vi "Example All Data.vi"() -> ()   [LabVIEW 2010]
uses:
  C:/tf/play/labview/Tinkerforge.dll
  Tinkerforge.dll
panel:
  out "calibration status":u8
  out "temperature (°C)":i16
  out "gravity vector (m/s²)":sgl[](array[numeric])
  out "linear acceleration (m/s²)":sgl[](array[numeric])
  out "euler angle (°)":sgl[](array[numeric])
  out "angular velocity (°/s)":sgl[](array[numeric])
  out "magnetic field (µT)":sgl[](array[numeric])
  out "quaternion":sgl[](array[numeric])
  out "acceleration (m/s²)":sgl[](array[numeric]) format="%.2f"
  in  "stop":bool
  in  "uid":string="Ron"
  in  "port":i32=4223
  in  "host":string="localhost"
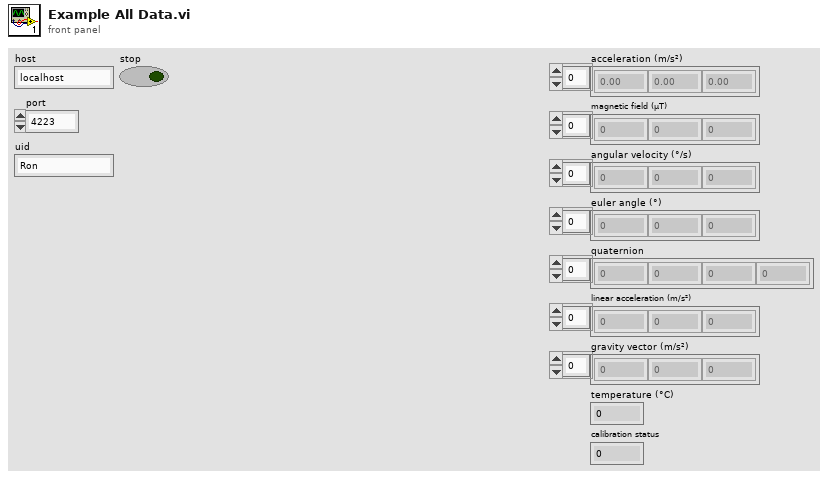
[diagram p1: front panel]
types:
  T1 = cluster{"acceleration":i16[], "magneticField":i16[], "angularVelocity":i16[], "eulerAngle":i16[], "quaternion":i16[], "linearAcceleration":i16[], "gravityVector":i16[], "temperature":i16, "calibrationStatus":u8}
  T2 = cluster{"acceleration[0]":i16, "acceleration[1]":i16, "acceleration[2]":i16, "acceleration[3]":i16, "acceleration[4]":i16, "acceleration[5]":i16, "acceleration[6]":i16, "acceleration[7]":i16, "acceleration[8]":i16}
  T3 = cluster{"magneticField[0]":i16, "magneticField[1]":i16, "magneticField[2]":i16, "magneticField[3]":i16, "magneticField[4]":i16, "magneticField[5]":i16, "magneticField[6]":i16, "magneticField[7]":i16, "magneticField[8]":i16}
  T4 = cluster{"angularVelocity[0]":i16, "angularVelocity[1]":i16, "angularVelocity[2]":i16, "angularVelocity[3]":i16, "angularVelocity[4]":i16, "angularVelocity[5]":i16, "angularVelocity[6]":i16, "angularVelocity[7]":i16, "angularVelocity[8]":i16}
  T5 = cluster{"eulerAngle[0]":i16, "eulerAngle[1]":i16, "eulerAngle[2]":i16, "eulerAngle[3]":i16, "eulerAngle[4]":i16, "eulerAngle[5]":i16, "eulerAngle[6]":i16, "eulerAngle[7]":i16, "eulerAngle[8]":i16}
  T6 = cluster{"quaternion[0]":i16, "quaternion[1]":i16, "quaternion[2]":i16, "quaternion[3]":i16, "quaternion[4]":i16, "quaternion[5]":i16, "quaternion[6]":i16, "quaternion[7]":i16, "quaternion[8]":i16}
  T7 = cluster{"linearAcceleration[0]":i16, "linearAcceleration[1]":i16, "linearAcceleration[2]":i16, "linearAcceleration[3]":i16, "linearAcceleration[4]":i16, "linearAcceleration[5]":i16, "linearAcceleration[6]":i16, "linearAcceleration[7]":i16, "linearAcceleration[8]":i16}
  T8 = cluster{"gravityVector[0]":i16, "gravityVector[1]":i16, "gravityVector[2]":i16, "gravityVector[3]":i16, "gravityVector[4]":i16, "gravityVector[5]":i16, "gravityVector[6]":i16, "gravityVector[7]":i16, "gravityVector[8]":i16}
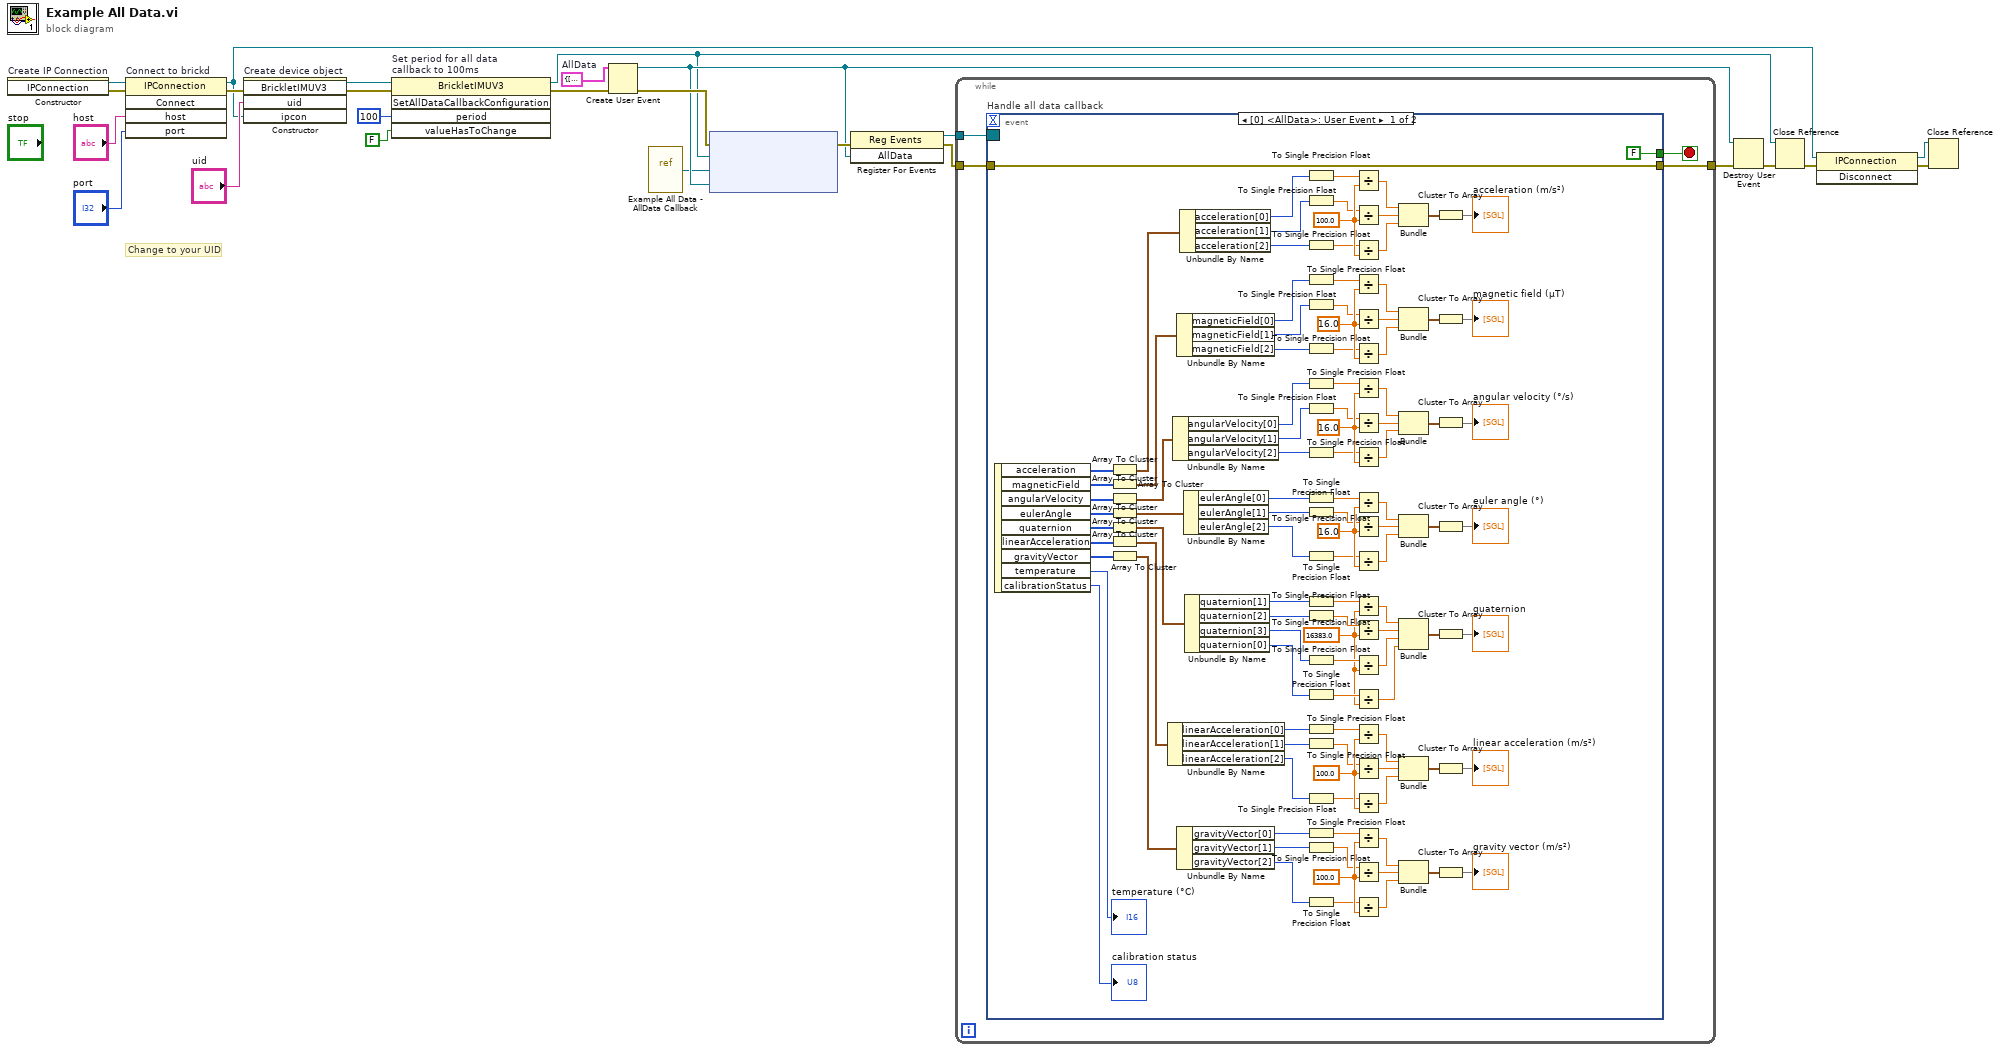
[diagram p0: block diagram]
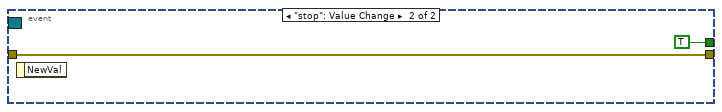
[diagram p2: hidden frame]
diagram:
  w9 = T1 {"acceleration"=[], "magneticField"=[], "angularVelocity"=[], "eulerAngle"=[], "quaternion"=[], "linearAcceleration"=[], "gravityVector"=[], "temperature"=0, "calibrationStatus"=0}  # AllData
  # "Change to your UID"
  n1 = constructor on="Create IP Connection" class="IPConnection"() -> (reference out=w25:refnum<k24>, error out=w3:errorcluster)  [unwired: 3 in, 1 out]
  n2 = invoke on="Connect to brickd" class="IPConnection" method="Connect"(reference=w25, error in=w3, "host"="host", "port"="port") -> (reference out=w18:refnum<k24>, error out=w21:errorcluster)  [unwired: 1 in, 3 out]
  n3 = constructor on="Create device object" class="BrickletIMUV3"(error in=w21, "uid"="uid", "ipcon"=w18) -> (reference out=w6:refnum<k24>, error out=w8:errorcluster)  [unwired: 2 in, 3 out]
  n4 = invoke on="Set period for all data\ncallback to 100ms" class="BrickletIMUV3" method="SetAllDataCallbackConfiguration"(reference=w6, error in=w8, "period"=i64 100, "valueHasToChange"=FALSE) -> (reference out=w5:refnum<k24>, error out=w7:errorcluster)  [unwired: 1 in, 3 out]
  n5 = Create User Event(user event datatype=w9, error in=w7) -> (user event=w11:refnum<user-event>, error out=w16:errorcluster)
  n6 = vi-ref "Example All Data - AllData Callback.vi"() -> ("vi reference"=w1:refnum<vi>)
  n7 = node ("Register Event Callback")(w16, w5, w1, w11) -> (w15:errorcluster)  [unwired: 1 in, 1 out]
  n8 = register-events(error in=w15, w11) -> (reference out=w14:refnum<event-registration>, error out=w12:errorcluster)  [unwired: 1 in]
  n9 = while {
    tunnel: w14 -> [w29]
    tunnel: [w28] -> w13
    tunnel: w12 -> [w27]
    stop <- w26 stop-if-true
    n10 = event "Handle all data callback" shown="[0] <AllData>: User Event" {
      selector: w29 -> [_ _]
      dyn-events: _ -> [_ _]
      timeout: _ -> [_ _]
      tunnel: [w134 w135] -> w28
      tunnel: w27 -> [w134 w135]
      tunnel: [FALSE TRUE] -> w26
      event User Event {
        w38 = sgl 100.0 ("y")
        w52 = sgl 100.0 ("y")
        w66 = sgl 16.0 ("y")
        w80 = sgl 16.0 ("y")
        w94 = sgl 16.0 ("y")
        w103 = sgl 16383.0 ("y")
        w123 = sgl 100.0 ("y")
        n11 = event-data() -> ("acceleration"=w132:i16[], "magneticField"=w89:i16[], "angularVelocity"=w75:i16[], "eulerAngle"=w60:i16[], "quaternion"=w107:i16[], "linearAcceleration"=w47:i16[], "gravityVector"=w33:i16[], "temperature"=→"temperature (°C)":i16, "calibrationStatus"=→"calibration status":u8)  [unwired: 1 in]
        n12 = Array To Cluster(array=w132) -> (cluster=w131:T2)
        n13 = Array To Cluster(array=w89) -> (cluster=w101:T3)
        n14 = Array To Cluster(array=w75) -> (cluster=w87:T4)
        n15 = Array To Cluster(array=w60) -> (cluster=w73:T5)
        n16 = Array To Cluster(array=w107) -> (cluster=w118:T6)
        n17 = Array To Cluster(array=w47) -> (cluster=w59:T7)
        n18 = Array To Cluster(array=w33) -> (cluster=w45:T8)
        n19 = Unbundle By Name(w59) -> ("linearAcceleration[0]"=w54:i16, "linearAcceleration[1]"=w51:i16, "linearAcceleration[2]"=w50:i16)
        n20 = Unbundle By Name(w87) -> ("angularVelocity[0]"=w82:i16, "angularVelocity[1]"=w79:i16, "angularVelocity[2]"=w78:i16)
        n21 = Unbundle By Name(w101) -> ("magneticField[0]"=w96:i16, "magneticField[1]"=w93:i16, "magneticField[2]"=w92:i16)
        n22 = Unbundle By Name(w45) -> ("gravityVector[0]"=w40:i16, "gravityVector[1]"=w37:i16, "gravityVector[2]"=w36:i16)
        n23 = Unbundle By Name(w131) -> ("acceleration[0]"=w125:i16, "acceleration[1]"=w122:i16, "acceleration[2]"=w121:i16)
        n24 = Unbundle By Name(w73) -> ("eulerAngle[0]"=w68:i16, "eulerAngle[1]"=w65:i16, "eulerAngle[2]"=w64:i16)
        n25 = Unbundle By Name(w118) -> ("quaternion[1]"=w113:i16, "quaternion[2]"=w111:i16, "quaternion[3]"=w110:i16, "quaternion[0]"=w104:i16)
        n26 = To Single Precision Float(number=w125) -> (single precision float=w124:sgl)
        n27 = To Single Precision Float(number=w122) -> (single precision float=w120:sgl)
        n28 = To Single Precision Float(number=w121) -> (single precision float=w119:sgl)
        n29 = To Single Precision Float(number=w96) -> (single precision float=w95:sgl)
        n30 = To Single Precision Float(number=w93) -> (single precision float=w91:sgl)
        n31 = To Single Precision Float(number=w92) -> (single precision float=w90:sgl)
        n32 = To Single Precision Float(number=w82) -> (single precision float=w81:sgl)
        n33 = To Single Precision Float(number=w79) -> (single precision float=w77:sgl)
        n34 = To Single Precision Float(number=w78) -> (single precision float=w76:sgl)
        n35 = To Single Precision Float(number=w68) -> (single precision float=w67:sgl)
        n36 = To Single Precision Float(number=w65) -> (single precision float=w63:sgl)
        n37 = To Single Precision Float(number=w64) -> (single precision float=w62:sgl)
        n38 = To Single Precision Float(number=w113) -> (single precision float=w112:sgl)
        n39 = To Single Precision Float(number=w111) -> (single precision float=w109:sgl)
        n40 = To Single Precision Float(number=w110) -> (single precision float=w108:sgl)
        n41 = To Single Precision Float(number=w104) -> (single precision float=w106:sgl)
        n42 = To Single Precision Float(number=w54) -> (single precision float=w53:sgl)
        n43 = To Single Precision Float(number=w51) -> (single precision float=w49:sgl)
        n44 = To Single Precision Float(number=w50) -> (single precision float=w48:sgl)
        n45 = To Single Precision Float(number=w40) -> (single precision float=w39:sgl)
        n46 = To Single Precision Float(number=w37) -> (single precision float=w35:sgl)
        n47 = To Single Precision Float(number=w36) -> (single precision float=w34:sgl)
        n48 = Divide(x=w124, y=w123) -> (x/y=w128:sgl)
        n49 = Divide(x=w120, y=w123) -> (x/y=w127:sgl)
        n50 = Divide(x=w119, y=w123) -> (x/y=w126:sgl)
        n51 = Divide(x=w95, y=w94) -> (x/y=w99:sgl)
        n52 = Divide(x=w91, y=w94) -> (x/y=w98:sgl)
        n53 = Divide(x=w90, y=w94) -> (x/y=w97:sgl)
        n54 = Divide(x=w81, y=w80) -> (x/y=w85:sgl)
        n55 = Divide(x=w77, y=w80) -> (x/y=w84:sgl)
        n56 = Divide(x=w76, y=w80) -> (x/y=w83:sgl)
        n57 = Divide(x=w67, y=w66) -> (x/y=w71:sgl)
        n58 = Divide(x=w63, y=w66) -> (x/y=w70:sgl)
        n59 = Divide(x=w62, y=w66) -> (x/y=w69:sgl)
        n60 = Divide(x=w112, y=w103) -> (x/y=w116:sgl)
        n61 = Divide(x=w109, y=w103) -> (x/y=w115:sgl)
        n62 = Divide(x=w108, y=w103) -> (x/y=w114:sgl)
        n63 = Divide(x=w106, y=w103) -> (x/y=w105:sgl)
        n64 = Divide(x=w53, y=w52) -> (x/y=w57:sgl)
        n65 = Divide(x=w49, y=w52) -> (x/y=w56:sgl)
        n66 = Divide(x=w48, y=w52) -> (x/y=w55:sgl)
        n67 = Divide(x=w39, y=w38) -> (x/y=w43:sgl)
        n68 = Divide(x=w35, y=w38) -> (x/y=w42:sgl)
        n69 = Divide(x=w34, y=w38) -> (x/y=w41:sgl)
        n70 = Bundle(w128, w127, w126) -> (w130:cluster{sgl, sgl, sgl})  [unwired: 1 in]
        n71 = Bundle(w99, w98, w97) -> (w100:cluster{sgl, sgl, sgl})  [unwired: 1 in]
        n72 = Bundle(w85, w84, w83) -> (w86:cluster{sgl, sgl, sgl})  [unwired: 1 in]
        n73 = Bundle(w71, w70, w69) -> (w72:cluster{sgl, sgl, sgl})  [unwired: 1 in]
        n74 = Bundle(w116, w115, w114, w105) -> (w117:cluster{sgl, sgl, sgl, sgl})  [unwired: 1 in]
        n75 = Bundle(w57, w56, w55) -> (w58:cluster{sgl, sgl, sgl})  [unwired: 1 in]
        n76 = Bundle(w43, w42, w41) -> (w44:cluster{sgl, sgl, sgl})  [unwired: 1 in]
        n77 = Cluster To Array(cluster=w130) -> (array=→"acceleration (m/s²)":sgl[])
        n78 = Cluster To Array(cluster=w100) -> (array=→"magnetic field (µT)":sgl[])
        n79 = Cluster To Array(cluster=w86) -> (array=→"angular velocity (°/s)":sgl[])
        n80 = Cluster To Array(cluster=w72) -> (array=→"euler angle (°)":sgl[])
        n81 = Cluster To Array(cluster=w117) -> (array=→"quaternion":sgl[])
        n82 = Cluster To Array(cluster=w58) -> (array=→"linear acceleration (m/s²)":sgl[])
        n83 = Cluster To Array(cluster=w44) -> (array=→"gravity vector (m/s²)":sgl[])
      }
      event "stop": Value Change {
        n84 = event-data() -> ()  [unwired: 1 in, 1 out]
      }
    }
  }
  n85 = Destroy User Event(user event=w11, error in=w13) -> (error out=w10:errorcluster)
  n86 = Close Reference(reference=w5, error in (no error)=w10) -> (error out=w20:errorcluster)
  n87 = invoke class="IPConnection" method="Disconnect"(reference=w18, error in=w20) -> (reference out=w17:refnum<k24>, error out=w19:errorcluster)  [unwired: 1 in, 1 out]
  n88 = Close Reference(reference=w17, error in (no error)=w19) -> ()  [unwired: 1 out]
